vi "Get IC.vi"(8 "error in (no error)":errorcluster, 10 "Domain":refnum<class "NI_Domain.lvclass">, 11 "IC_1D_Numeric in":refnum<class "NI_IC_1D_Numeric.lvclass">) -> (0 "error out":errorcluster, 2 "IC":variant, 3 "IC_1D_Numeric out":refnum<class "NI_IC_1D_Numeric.lvclass">)   [LabVIEW 2020, in "NI_PDE.lvlib" / "NI_IC_1D_Numeric.lvclass"]
uses:
  <vilib>/gmath/pde.llb/ICClass/IC_1D_Numeric/NI_IC_1D_Numeric.lvclass
  <vilib>/gmath/pde.llb/DomainClass/NI_Domain.lvclass
  <vilib>/gmath/pde.llb/ICClass/IC_1D_Numeric/IC Data.ctl
  <vilib>/gmath/pde.llb/Common/PDE_IC Type.ctl
  <vilib>/gmath/pde.llb/ICClass/IC_1D_Numeric/NI_IC_1D_Numeric.lvclass/NI_IC_1D_Numeric.ctl
  <vilib>/gmath/NI_PDE.lvlib
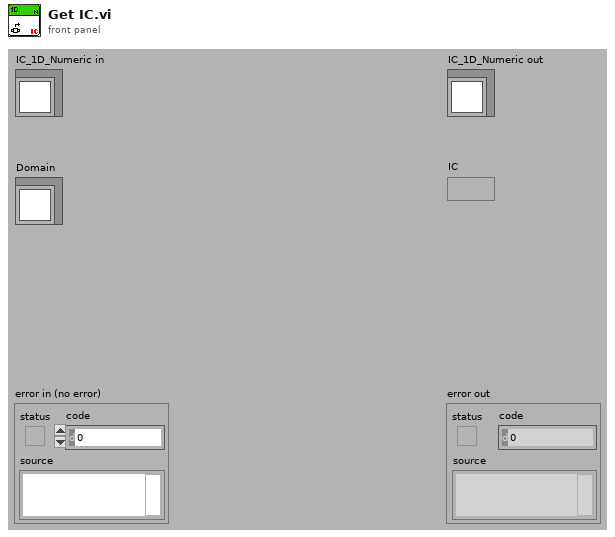
[diagram p1: front panel]
types:
  T1 = typedef "NI_PDE.lvlib/NI_IC_1D_Numeric.lvclass/IC Data.ctl" = cluster{"type":T2, "H":dbl[]}
  T2 = typedef "NI_PDE.lvlib/PDE_IC Type.ctl" = i32
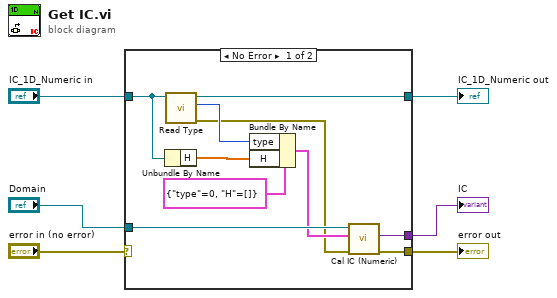
[diagram p0: block diagram]
diagram:
  n1 = case shown="No Error" "error in (no error)" {
    selector: "error in (no error)" -> [_ w18]
    tunnel: "IC_1D_Numeric in" -> [w7 w17]
    tunnel: "Domain" -> [w13 _]
    tunnel: [w10 w18] -> w4
    tunnel: [w9 _] -> w3
    tunnel: [w16 w17] -> w2
    frame No Error {
      n2 = Unbundle By Name(w7) -> ("H"=w8:dbl[])
      n3 = call-dynamic "Read Type.vi"("IC.lvclass in"=w7) -> ("error out"=w11:errorcluster, "IC type"=w14:T2, "IC.lvclass out"=w16:refnum<class "NI_IC_1D_Numeric.lvclass">)  [unwired: 1 in, 7 out]
      n4 = Bundle By Name(cluster=T1 {"type"=0, "H"=[]} ("IC data"), "type"=w14, "H"=w8) -> (w12:T1)
      n5 = call-dynamic "Cal IC (Numeric).vi"("error in (no error)"=w11, "IC in"=w12, "Domain in"=w13) -> ("error out"=w10:errorcluster, "IC out"=w9:variant)  [unwired: 7 out]
    }
    frame Error {
    }
  }
  "IC" <- w3
  "error out" <- w4
  "IC_1D_Numeric out" <- w2
